vi "test_conv.vi"() -> ()   [LabVIEW 2018]
uses:
  <vilib>/Analysis/1siggen.llb/Ramp Pattern by Samples.vi
  <vilib>/addons/Modulation/Digital/General/MT Generate Bits (Galois, PN Order).vi
  <vilib>/addons/Modulation/Digital/Channel Coding/MT Convolutional Encoder (Rate).vi
  <vilib>/Analysis/baseanly.llb/Mean (DBL).vi
  <vilib>/addons/Modulation/Analog/support/mod_Set Error Source.vi
  <vilib>/addons/Modulation/Digital/Support/Common/Validators/mod_Generate Bits Validate.vi
  <vilib>/addons/Modulation/Digital/Support/Common/Validators/mod_Validate Bit Stream.vi
  <vilib>/addons/Modulation/Digital/Channel Coding/Convolutional codes/mod_Convolutional encoder.vi
  <vilib>/addons/Modulation/Digital/Support/Common/Validators/mod_AWGN Validate.vi
  <vilib>/addons/Modulation/Digital/Impairments/subVIs/mod_createSeeds.vi
  <vilib>/addons/Modulation/Digital/Channel Coding/Convolutional codes/subVIs/mod_Generate encoder tap connections.vi
  <vilib>/addons/Modulation/Digital/Channel Coding/Convolutional codes/subVIs/mod_Perform convolutional encoding.vi
  <vilib>/addons/Modulation/Digital/Channel Coding/Block codes/subVIs/mod_Buffer block code info (I8).vi
  <vilib>/addons/Modulation/Digital/Channel Coding/Convolutional codes/subVIs/mod_Generate valid reset (convolutional, I8).vi
  <vilib>/addons/Modulation/Digital/Support/Common/Validators/mod_Validate Samples Per Symbol.vi
  <vilib>/addons/Modulation/Analog/support/Validators/mod_Validate Complex Waveform.vi
  <vilib>/addons/Modulation/Analog/support/Validators/mod_WFErrorHandler.vi
  <vilib>/addons/Modulation/Digital/Support/Common/Validators/mod_Generate Filter Coefficients Validate.vi
  <vilib>/addons/Modulation/Digital/General/subVIs/mod_Generate Filter Coefficients.vi
  <vilib>/addons/Modulation/Digital/General/MT Generate PSK System Parameters(M).vi
  <vilib>/addons/Modulation/Digital/General/subVIs/mod_Generate Bits PN Sequence.vi
  <vilib>/addons/Modulation/Digital/Channel Coding/Convolutional codes/subVIs/mod_Select known generator matrix.vi
  <vilib>/addons/Modulation/Digital/Support/Common/Validators/mod_Validate Convolutional Encoder prms.vi
  <vilib>/Analysis/1siggen.llb/Gaussian White Noise (obs 90).vi
  <vilib>/addons/Modulation/Digital/General/MT Apply Matched Filter (Generic).vi
  <vilib>/addons/Modulation/Digital/General/MT Map PSK Symbols to Bits.vi
  <vilib>/addons/Modulation/Digital/Channel Coding/MT Convolutional Decoder (Viterbi Hard Decision, Rate).vi
  <vilib>/addons/Modulation/Digital/Demodulation/MT Calculate BER After Trigger (PN Sequence).vi
  <vilib>/addons/Modulation/niDMT.lvlib
  <vilib>/Analysis/NI_AALBase.lvlib
panel:
  out "output bit stream":i8[](array[numeric])
  out "mess_codé":i8[](array[numeric])
  out "size(s) 3":i32
  out "message":i8[](array[numeric])
  out "size(s) 2":i32
  out "size(s)":i32
  out "out_perso":i8[](array[numeric])
  out "Y":cdb[](array[numeric])
  out "IQ Constellation":T1(graph)
  in  "Traceback Depth (D)":i32=20
  in  "Constraint Length (K)":i32=3
  in  "Rate (k/n)":enum16{"1/2", "1/3", "1/4", "2/3", "3/4"}(ring)
  in  "PN Sequence Order":i32=19
  in  "Seed In":i32=-1
  out "BER vs Eb/N0 (dB)\n[AWGN channel]":cluster{"Ramp Pattern":dbl[], dbl[]}(graph)
  in  "Trials per Eb/N0 Sample":i32=1
  in  "Start Eb/N0 (dB)":dbl=5.0 format="%0.2f"
  in  "End Eb/N0 (dB)":dbl=10.0 format="%0.2f"
  in  "Eb/N0 Samples":i32=6
  out "Progress in current trial":i32(slide) scale=0.0..100.0
  out "Accumulated BER (coding)":dbl format="%.4p"
  out "Current trial":i32
  out "Current Eb/N0":dbl
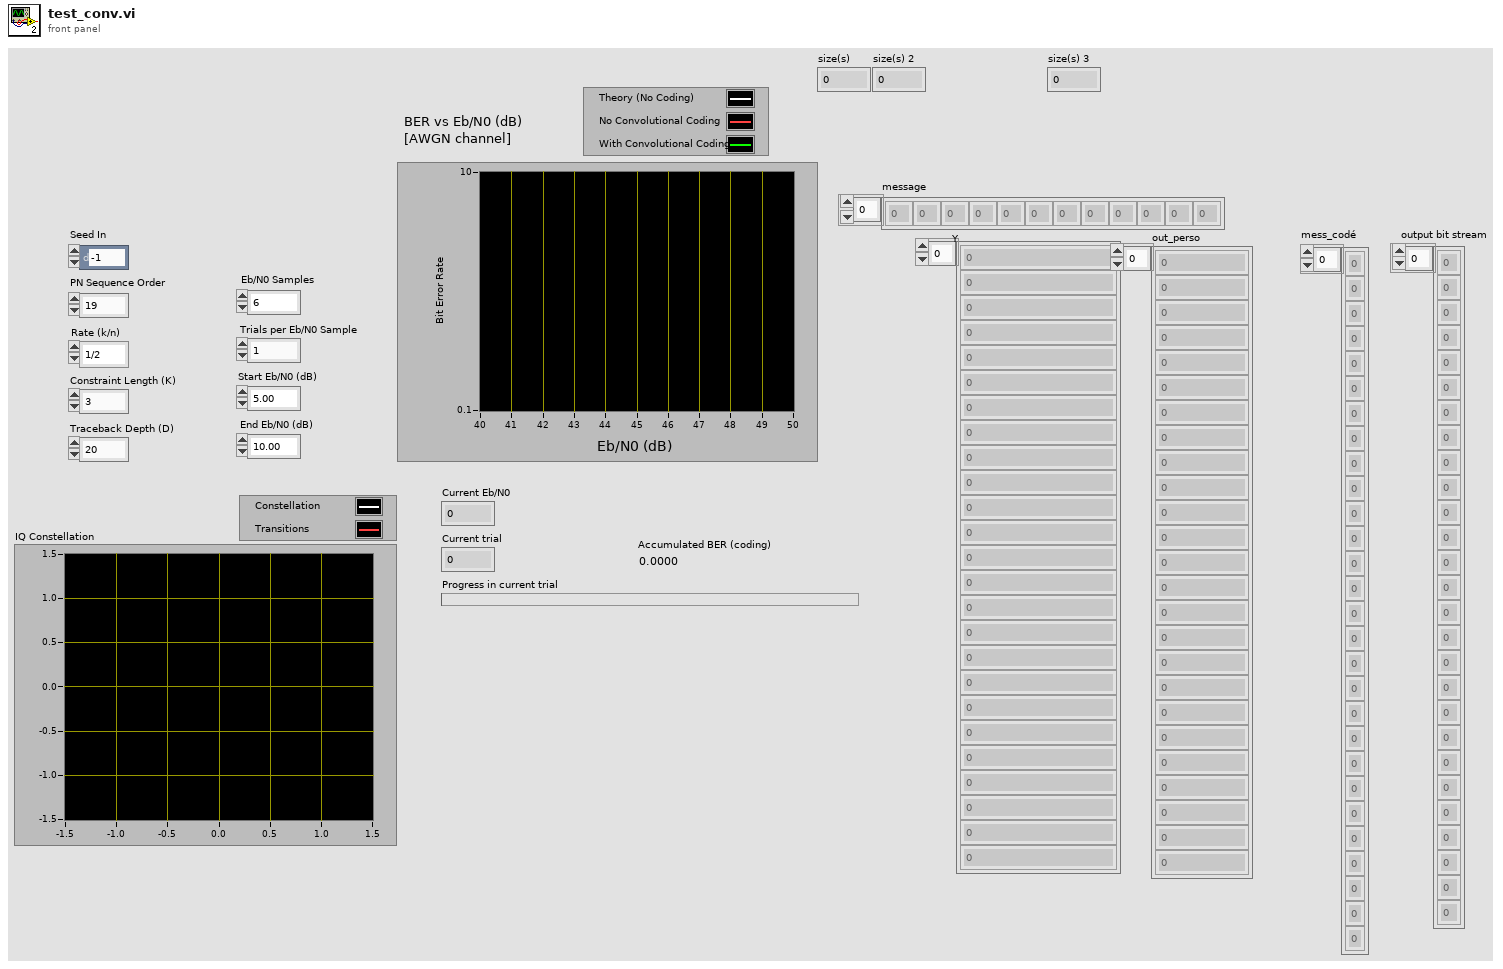
[diagram p1: front panel]
types:
  T1 = cluster{"Decimated Array":dbl[], "Decimated Array":dbl[]}[]
  T2 = enum16{"none", "Raised Cosine", "Root Raised Cos", "Gaussian"}
  T3 = cluster{"samples per symbol (16)":i32, "symbol map":cdb[], "differential PSK":enum16{"disable", "enable"}, "PSK type":u16}
  T4 = typedef "niAMT.lvlib/Complex Data Waveform.ctl" = cluster{"t0":dbl, "dt":dbl, "Y":cdb[]}
  T5 = cluster{"constellation":dbl[], "oversampled data":dbl[]}[]
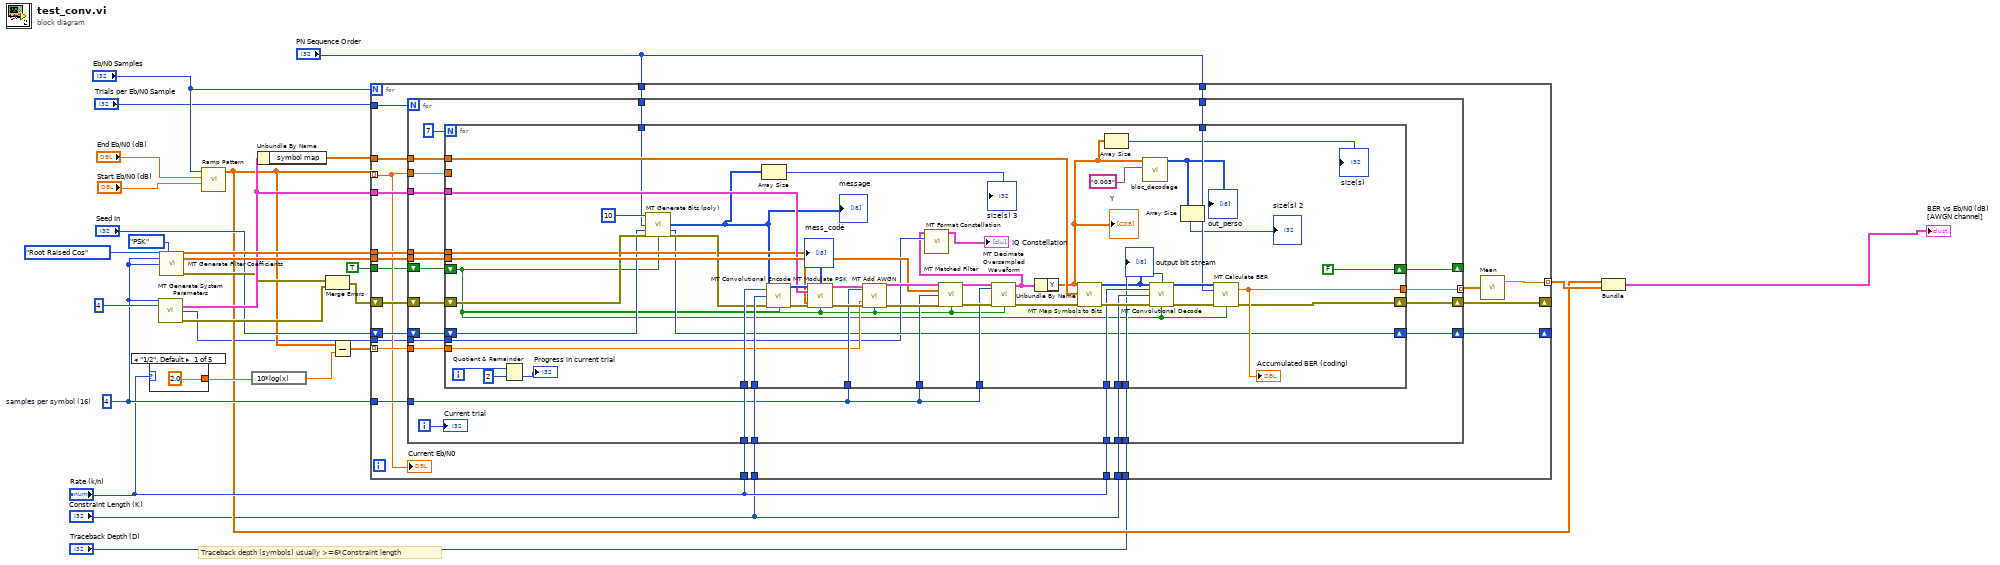
[diagram p0: block diagram]
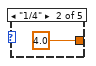
[diagram p2: hidden frame]
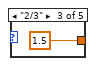
[diagram p3: hidden frame]
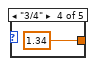
[diagram p4: hidden frame]
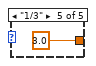
[diagram p5: hidden frame]
diagram:
  w21 = 4  # samples per symbol (16)
  # "Traceback depth (symbols) usually >=6*Constraint length"
  n1 = case shown="\"1/2\", Default" "Rate (k/n)" {
    tunnel: [2.0 4.0 1.5 1.34 3.0] -> w8
    frame "1/2", Default {
    }
    frame "1/4" {
    }
    frame "2/3" {
    }
    frame "3/4" {
    }
    frame "1/3" {
    }
  }
  n2 = call-poly <vilib>:"MT Generate System Parameters.vi"("samples per symbol (16)"=w21, "M-PSK (4)"=4) -> ("PSK system parameters"=w20:T3, "bits per symbol"=w2:i32, "error out"=w15:errorcluster)  [unwired: 11 in]
  n3 = call <vilib>:"MT Generate Filter Coefficients.vi"("pulse shaping filter (none)"=T2."Root Raised Cos", "modulation type"=enum16{"FSK", "PSK", "QAM", "MSK", "PAM", "ASK"}."PSK", "pulse shaping samples per symbol (16)"=w21, "matched samples per symbol (16)"=w21) -> ("pulse shaping filter coefficients"=w26:dbl[], "matched filter coefficients"=w22:dbl[], "error out"=w16:errorcluster)  [unwired: 9 in]
  n4 = call-poly <vilib>:"Ramp Pattern.vi"("start"="Start Eb/N0 (dB)", "end"="End Eb/N0 (dB)", "samples"="Eb/N0 Samples") -> ("Ramp Pattern"=w6:dbl[])  [unwired: 7 in, 1 out]
  n5 = expression code="10*log(x)"(w8) -> (w7:dbl)
  n6 = Unbundle By Name(w20) -> ("symbol map"=w19:cdb[])
  n7 = Merge Errors(w16, w15) -> (w14:errorcluster)
  n8 = Subtract(x=w6, y=w7) -> (x-y=w13:dbl[])
  n9 = for {
    N: "Eb/N0 Samples" -> [_]
    tunnel: w26 -> [w56]
    tunnel: "Rate (k/n)" -> [w54]
    tunnel: "Constraint Length (K)" -> [w53]
    tunnel: w6 -> [w36] mode=indexing
    tunnel: w22 -> [w52]
    tunnel: w21 -> [w51]
    tunnel: w19 -> [w50]
    tunnel: "Rate (k/n)" -> [w49]
    tunnel: "Constraint Length (K)" -> [w48]
    tunnel: "Traceback Depth (D)" -> [w47]
    tunnel: "Trials per Eb/N0 Sample" -> [w46]
    tunnel: [w44] -> w10 mode=indexing
    tunnel: w20 -> [w55]
    shift-right: [w43] -> _
    shift-left: w14 -> [w42]
    tunnel: w13 -> [w41] mode=indexing
    shift-right: [w39] -> _
    shift-left: "Seed In" -> [w40]
    tunnel: "PN Sequence Order" -> [w38]
    tunnel: "PN Sequence Order" -> [w37]
    tunnel: TRUE ("reset? (T)") -> [w35]
    tunnel: w2 -> [w34]
    n10 = for {
      N: w46 -> [_]
      tunnel: w56 -> [w80]
      tunnel: w54 -> [w78]
      tunnel: w53 -> [w77]
      tunnel: w36 -> [w76]
      tunnel: w52 -> [w75]
      tunnel: w51 -> [w74]
      tunnel: w50 -> [w73]
      tunnel: w49 -> [w72]
      tunnel: w48 -> [w71]
      tunnel: w47 -> [w70]
      tunnel: [w68] -> w45 mode=indexing
      tunnel: w55 -> [w79]
      shift-right: [w66] -> w43
      shift-left: w42 -> [w65]
      tunnel: w41 -> [w64]
      shift-right: [w62] -> w39
      shift-left: w40 -> [w63]
      tunnel: w38 -> [w61]
      tunnel: w37 -> [w60]
      shift-right: [w58] -> _
      shift-left: w35 -> [w59]
      tunnel: w34 -> [w57]
      i -> [w67]
      n11 = for {
        N: 7 -> [_]
        tunnel: w80 -> [w103]
        shift-right: [FALSE ("reset? (T)")] -> w58
        shift-left: w59 -> [w81]
        tunnel: w78 -> [w128]
        tunnel: w77 -> [w127]
        tunnel: w76 -> [_]
        tunnel: w75 -> [w124]
        tunnel: w74 -> [w118]
        tunnel: w74 -> [w116]
        tunnel: w74 -> [w117]
        tunnel: w73 -> [w114]
        tunnel: w72 -> [w112]
        tunnel: w71 -> [w111]
        tunnel: w70 -> [w110]
        tunnel: [w106] -> w68
        tunnel: w79 -> [w121]
        shift-right: [w92] -> w66
        shift-left: w65 -> [w105]
        tunnel: w64 -> [w102]
        shift-right: [w100] -> w62
        shift-left: w63 -> [w101]
        tunnel: w61 -> [w99]
        tunnel: w60 -> [w98]
        tunnel: w57 -> [w93]
        i -> [w96]
        n12 = Quotient & Remainder(x=w96, y=2) -> (floor(x/y)=→"Progress in current trial":i32)  [unwired: 1 out]
        n13 = call-poly <vilib>:"MT Generate Bits (poly).vi"("total bits (128)"=10, "PN sequence order (9)"=w99, "seed in (0xD6BF7DF2)"=w101, "error in (no error)"=w105, "reset? (T)"=w81) -> ("output bit stream"=w83:i8[], "seed out"=w100:i32, "error out"=w104:errorcluster)  [unwired: 8 in]
        "message" <- w83
        n14 = Array Size(array=w83) -> (size(s)=→"size(s) 3":i32)
        n15 = call-poly <vilib>:"MT Convolutional Encode.vi"("input bit stream"=w83, "rate (k/n)"=w128, "constraint length (K)"=w127, "error in (no error)"=w104, "reset? (T)"=w81) -> ("output bit stream"=w129:i8[], "error out"=w122:errorcluster)  [unwired: 8 in, 1 out]
        "mess_codé" <- w129
        n16 = call <vilib>:"MT Modulate PSK.vi"("input bit stream"=w129, "PSK system parameters"=w121, "pulse shaping filter coefficients"=w103, "error in (no error)"=w122, "reset? (T)"=w81) -> ("output complex waveform"=w94:T4, "error out"=w123:errorcluster)  [unwired: 8 in, 1 out]
        n17 = call <vilib>:"MT Add AWGN.vi"("input complex waveform"=w94, "samples per symbol (16)"=w117, "Eb/N0 (10 dB)"=w102, "error in (no error)"=w123, "reset? (T)"=w81) -> ("output complex waveform"=w125:T4, "error out"=w126:errorcluster)  [unwired: 8 in, 1 out]
        n18 = call-poly <vilib>:"MT Matched Filter.vi"("input complex waveform"=w125, "matched filter coefficients"=w124, "samples per symbol (16)"=w116, "error in (no error)"=w126, "reset? (T)"=w81) -> ("output complex waveform"=w120:T4, "error out"=w119:errorcluster)  [unwired: 9 in]
        n19 = call <vilib>:"MT Decimate Oversampled Waveform.vi"("input complex waveform"=w120, "decimation factor"=w118, "error in (no error)"=w119, "reset? (T)"=w81) -> ("output complex waveform"=w91:T4, "error out"=w115:errorcluster)  [unwired: 10 in]
        n20 = call <vilib>:"MT Format Constellation.vi"("waveform"=w91, "samples per symbol"=w93) -> ("constellation graph"=→"IQ Constellation":T5)  [unwired: 12 in, 1 out]
        n21 = Unbundle By Name(w91) -> ("Y"=w87:cdb[])
        "Y" <- w87
        n22 = call-poly <vilib>:"MT Map Symbols to Bits.vi"("symbols"=w87, "symbol map"=w114, "error in (no error)"=w115) -> ("output bit stream"=w89:i8[], "error out"=w113:errorcluster)  [unwired: 11 in]
        "output bit stream" <- w89
        n23 = Array Size(array=w87) -> (size(s)=→"size(s)":i32)
        n24 = call "bloc_decodage.vi"("sigma2"="0.003", "Array"=w87) -> ("output bit stream"=w84:i8[])  [unwired: 7 in, 2 out]
        "out_perso" <- w84
        n25 = call-poly <vilib>:"MT Convolutional Decode.vi"("input bit stream"=w89, "traceback depth (D)"=w110, "rate (k/n)"=w112, "constraint length (K)"=w111, "error in (no error)"=w113, "reset? (T)"=w81) -> ("output bit stream"=w108:i8[], "error out"=w109:errorcluster)  [unwired: 7 in, 1 out]
        n26 = Array Size(array=w84) -> (size(s)=→"size(s) 2":i32)
        n27 = call-poly <vilib>:"MT Calculate BER.vi"("input bit stream"=w108, "PN sequence order (9)"=w98, "error in (no error)"=w109, "reset? (T)"=w81) -> ("accumulated BER"=w106:dbl, "error out"=w92:errorcluster)  [unwired: 7 in, 3 out]
        "Accumulated BER (coding)" <- w106
      }
      "Current trial" <- w67
    }
    n28 = call-poly <vilib>:"Mean.vi"("X"=w45) -> ("mean"=w44:dbl)  [unwired: 1 out]
    "Current Eb/N0" <- w36
  }
  n29 = Bundle("Ramp Pattern"=w6, w10) -> (→"BER vs Eb/N0 (dB)\n[AWGN channel]":cluster{"Ramp Pattern":dbl[], dbl[]})  [unwired: 1 in]
